vi "Do.vi"(8 "error in (no error)":errorcluster, 10 "Actor in":refnum<class "Simple Actor.lvclass">, 11 "Actor Msg in":refnum<class "Actor Msg.lvclass">) -> (0 "error out":errorcluster, 2 "Actor out":refnum<class "Simple Actor.lvclass">, 3 "Actor Msg out":refnum<class "Actor Msg.lvclass">)   [LabVIEW 2020, in "Simple Actor.lvlib" / "Actor Msg.lvclass"]
uses:
  Actor Msg.lvclass
  Simple Actor/Simple Actor.lvclass
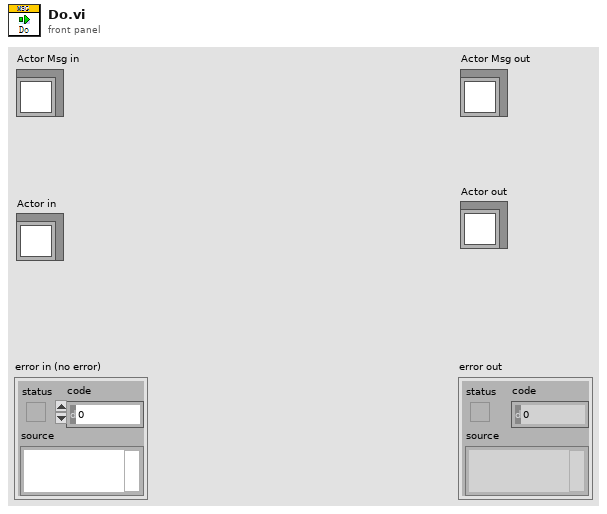
[diagram p1: front panel]
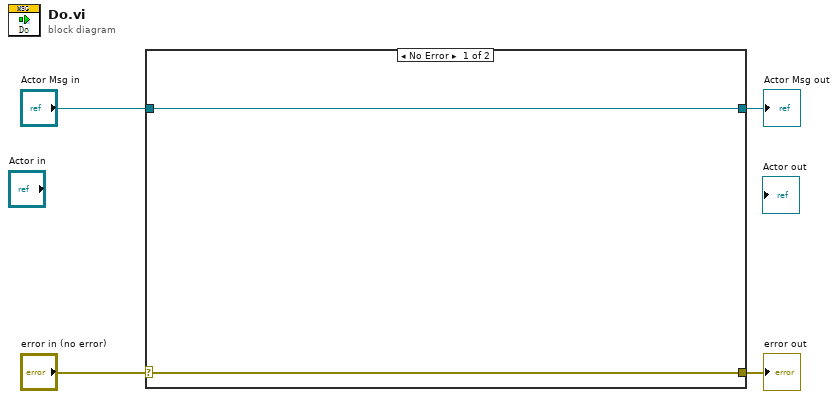
[diagram p0: block diagram]
diagram:
  n1 = case shown="No Error" "error in (no error)" {
    selector: "error in (no error)" -> [w5 w8]
    tunnel: [w5 w8] -> w3
    tunnel: [w6 w7] -> w1
    tunnel: "Actor Msg in" -> [w6 w7]
    frame No Error {
    }
    frame Error {
    }
  }
  "error out" <- w3
  "Actor Msg out" <- w1
